vi "Get Stop Event.vi"(8 "error in (no error)":errorcluster, 11 "Observable Actor in":refnum<class "Observable Actor.lvclass">) -> (0 "error out":errorcluster, 2 "Events":refnum<event-registration>, 3 "Observable Actor out":refnum<class "Observable Actor.lvclass">)   [LabVIEW 2014, in "Observable Actor.lvlib" / "Observable Actor.lvclass"]
uses:
  Observable Actor.lvclass
  Observable Actor.lvclass/Observable Actor.ctl
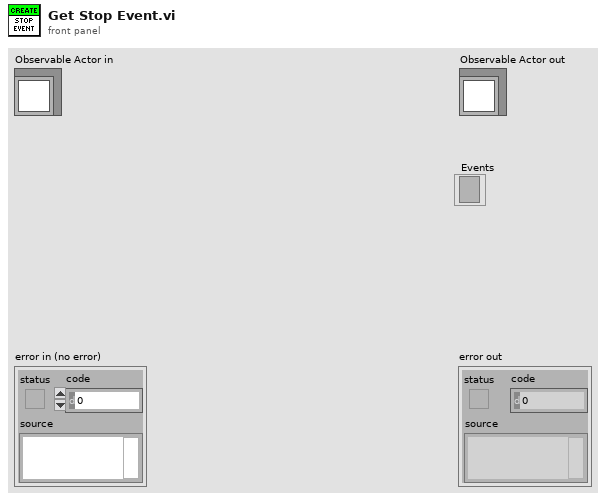
[diagram p1: front panel]
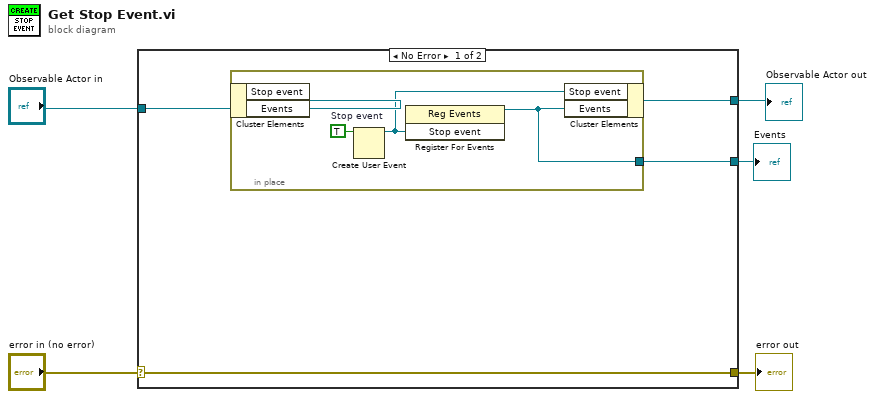
[diagram p0: block diagram]
diagram:
  n1 = case shown="No Error" "error in (no error)" {
    selector: "error in (no error)" -> [w9 w14]
    tunnel: [w9 w14] -> w4
    tunnel: [w7 w13] -> w1
    tunnel: "Observable Actor in" -> [w8 w13]
    tunnel: [w6 _] -> w3
    frame No Error {
      n2 = in-place {
        in-place-border: [w10] -> w6
        w12 = TRUE  # Stop event
        n3 = in-place-cluster #1(w8) -> ()  [unwired: 2 out]
        n4 = Create User Event(user event datatype=w12) -> (user event=w11:refnum<user-event>)  [unwired: 1 in, 1 out]
        n5 = register-events(w11) -> (reference out=w10:refnum<event-registration>)  [unwired: 2 in, 1 out]
        n6 = in-place-cluster #1("Stop event"=w11, "Events"=w10) -> (w7:refnum<class "Observable Actor.lvclass">)
      }
    }
    frame Error {
    }
  }
  "error out" <- w4
  "Events" <- w3
  "Observable Actor out" <- w1
